vi "parse_point_field.vi"(4 "error in":errorcluster, 7 "msg in":string) -> (0 "error out":errorcluster, 1 "PointField":T1, 2 "Header":T2, 3 "msg out":string)   [LabVIEW 2016]
uses:
  std_msgs/subs/parse_string_scalar.vi
  std_msgs/subs/parse_u32_scalar.vi
  std_msgs/subs/parse_u8_scalar.vi
panel:
  # "Datatype\nuint8 INT8    = 1\nuint8 UINT8   = 2\nuint8 INT16   = 3\nuint8 UINT16  = 4\nuint8 INT32   = 5\nuint8 UINT32  = 6\nuint8 FLOAT32 = 7\nuint8 FLOAT64 = 8"
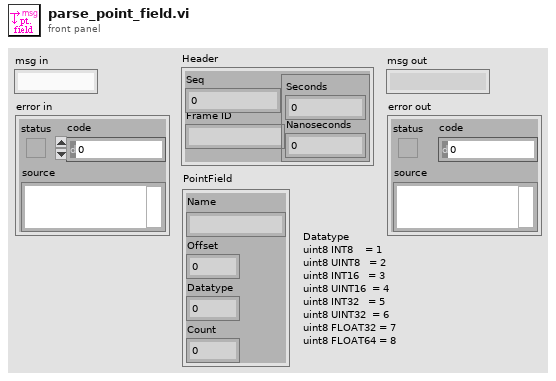
[diagram p1: front panel]
types:
  T1 = cluster{"Name":string, "Offset":u32, "Datatype":u8, "Count":u32}
  T2 = cluster{"Seq":u32, "Frame ID":string, cluster{"Seconds":i32, "Nanoseconds":i32}}
  T3 = cluster{"Seq":u32, "Frame ID":string, "Timestamp":cluster{"Seconds":i32, "Nanoseconds":i32}}
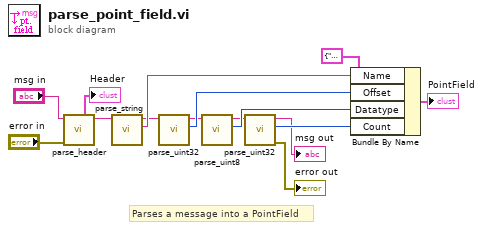
[diagram p0: block diagram]
diagram:
  # "Parses a message into a PointField"
  n1 = call "parse_header.vi"("error in"="error in", "msg in"="msg in") -> ("Header"=→"Header":T3, "msg out"=w11:string)  [unwired: 3 in, 1 out]
  n2 = call-poly "parse_string.vi"("msg in"=w11) -> ("string"=w12:string, "msg out"=w3:string)  [unwired: 4 in, 1 out]
  n3 = call-poly "parse_uint32.vi"("msg in"=w3) -> ("number"=w8:u32, "msg out"=w4:string)  [unwired: 4 in, 1 out]
  n4 = call-poly "parse_uint8.vi"("msg in"=w4) -> ("number"=w7:u8, "msg out"=w5:string)  [unwired: 4 in, 1 out]
  n5 = call-poly "parse_uint32.vi"("msg in"=w5) -> ("error out"=→"error out":errorcluster, "number"=w6:u32, "msg out"=→"msg out":string)  [unwired: 4 in]
  n6 = Bundle By Name(cluster=T1 {"Name"="", "Offset"=0, "Datatype"=0, "Count"=0} ("PointField"), "Name"=w12, "Offset"=w8, "Datatype"=w7, "Count"=w6) -> (→"PointField":T1)
